vi "Waveform Envelope.vi"() -> ()   [LabVIEW 2020]
panel:
  out "From Origin":dynamicdata(graph)
  in  "Visible":i32(ring) items=["MAINWND_HIDE"=0, "MAINWND_SHOW"=1, "MAINWND_SHOWMINIMIZED"=2, "MAINWND_SHOWMAXIMIZED"=3, "MAINWND_SHOW_BRING_TO_FRONT"=100]
  out "data filepath":path
  in  "GetEnvelope":bool
  out "ogw path":path
  out "Origin ogw Load":bool
  out "Error Out":errorcluster
  out "Input Data":waveform(dbl)(graph)
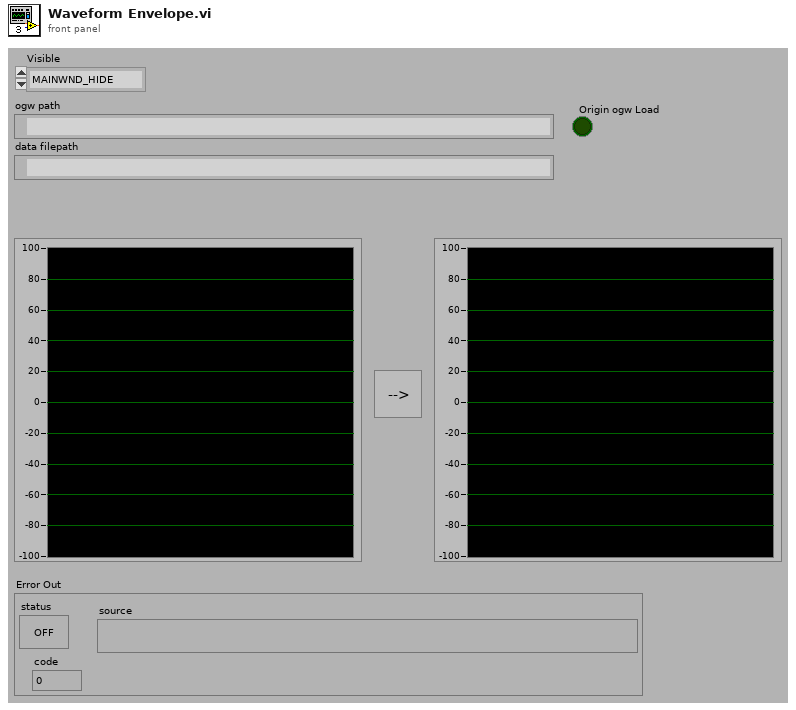
[diagram p1: front panel]
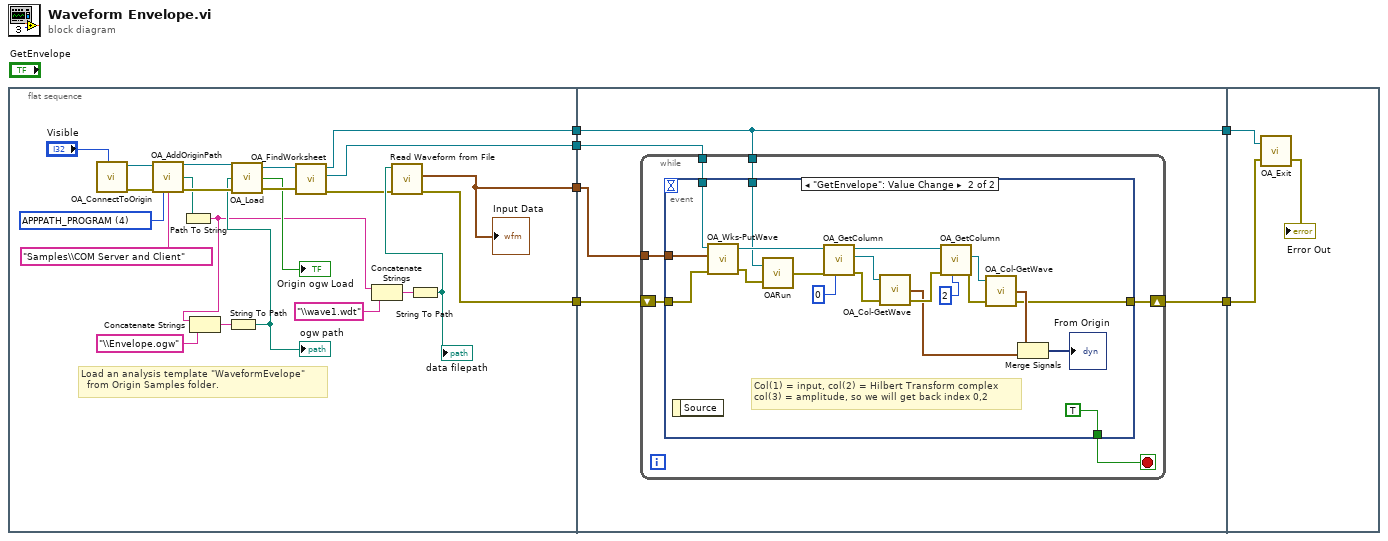
[diagram p0: block diagram]
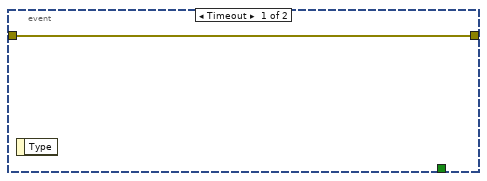
[diagram p2: hidden frame]
diagram:
  n1 = flat-sequence {
    tunnel: [w10] -> w6
    tunnel: [w9] -> w5
    tunnel: [w8] -> w4
    tunnel: [w7] -> w2
    tunnel: w6 -> [w34]
    tunnel: w5 -> [w32]
    tunnel: w4 -> [w33]
    tunnel: [w32] -> w3
    tunnel: w2 -> [w31]
    tunnel: [w30] -> w1
    tunnel: w3 -> [w63]
    tunnel: w1 -> [w62]
    frame #0 {
      w27 = 4 items=["APPPATH_USER"=2, "APPPATH_GROUP"=3, "APPPATH_PROGRAM"=4] ("Type")
      # "Load an analysis template \"WaveformEvelope\"\n  from Origin Samples folder."
      n2 = call "OA_ConnectToOrigin.vi"("Visible"="Visible") -> ("error out"=w22:errorcluster, "Origin.IOApplication"=w23:refnum<k7>)  [unwired: 7 in]
      n3 = call "OA_AddOriginPath.vi"("Origin.IOApplication"=w23, "error in (no error)"=w22, "Type"=w27, "Filename"="Samples\\COM Server and Client") -> ("Origin.IOApplication"=w29:refnum<k7>, "path out"=w17:path, "error out"=w28:errorcluster)  [unwired: 9 in]
      n4 = Path To String(path=w17) -> (string=w11:string)
      n5 = Concatenate Strings(w11, "\\Envelope.ogw" ("string")) -> (w19:string)
      n6 = String To Path(string=w19) -> (path=w18:path)
      "ogw path" <- w18
      n7 = call "OA_Load.vi"("error in (no error)"=w28, "Path"=w18, "Origin.IOApplication"=w29) -> ("error out"=w24:errorcluster, "Load"=→"Origin ogw Load":bool, "Origin.IOApplication"=w25:refnum<k7>)
      n8 = call "OA_FindWorksheet.vi"("error in (no error)"=w24, "Origin.IOApplication"=w25) -> ("error out"=w12:errorcluster, "Origin.Worksheet"=w8:refnum<k7>, "Origin.IOApplication"=w9:refnum<k7>)  [unwired: 7 in]
      n9 = Concatenate Strings(w11, "\\wave1.wdt" ("string")) -> (w14:string)
      n10 = String To Path(string=w14) -> (path=w15:path)
      "data filepath" <- w15
      n11 = call <vilib>:"Read Waveform from File.vi"("error in (no error)"=w12, "file path (dialog if empty)"=w15) -> ("error out"=w7:errorcluster, "first waveform in record"=w10:waveform(dbl))  [unwired: 4 in, 2 out]
      "Input Data" <- w10
    }
    frame #1 {
      n12 = while {
        tunnel: w34 -> [w40]
        tunnel: w33 -> [w39]
        tunnel: w32 -> [w38]
        shift-right: [w36] -> w30
        shift-left: w31 -> [w37]
        stop <- w35 stop-if-true
        n13 = event shown="[1] \"GetEnvelope\": Value Change" {
          selector: _ -> [_ _]
          dyn-events: _ -> [_ _]
          timeout: _ -> [_ _]
          tunnel: w40 -> [_ w49]
          tunnel: w39 -> [_ w48]
          tunnel: w38 -> [_ w47]
          tunnel: w37 -> [w41 w46]
          tunnel: [w41 w42] -> w36
          tunnel: [_ TRUE] -> w35
          event Timeout {
            n14 = event-data() -> ()  [unwired: 1 in, 1 out]
          }
          event "GetEnvelope": Value Change {
            # "Col(1) = input, col(2) = Hilbert Transform complex\ncol(3) = amplitude, so we will get back index 0,2"
            n15 = event-data() -> ()  [unwired: 1 in, 1 out]
            n16 = call "OA_Wks-PutWave.vi"("Origin.Worksheet"=w48, "Dynamic Data"=w49, "error in (no error)"=w46) -> ("Origin.Worksheet dup"=w59:refnum<k7>, "error IO"=w60:errorcluster)  [unwired: 3 in]
            n17 = call "OARun.vi"("Origin.IOApplication"=w47, "Error IO"=w60) -> ("Error IO Out"=w61:errorcluster)  [unwired: 2 out]
            n18 = call "OA_GetColumn.vi"("Column Name/Index"=0, "error in (no error)"=w61, "Origin.Worksheet"=w59) -> ("error out"=w56:errorcluster, "Origin.Column"=w43:refnum<k7>, "Origin.Worksheet"=w50:refnum<k7>)  [unwired: 6 in]
            n19 = call "OA_Col-GetWave.vi"("error in (no error)"=w56, "Origin.Column"=w43) -> ("error out"=w53:errorcluster, "Waveform Out"=w52:waveform(dbl))  [unwired: 1 in, 1 out]
            n20 = call "OA_GetColumn.vi"("Column Name/Index"=2, "error in (no error)"=w53, "Origin.Worksheet"=w50) -> ("error out"=w54:errorcluster, "Origin.Column"=w55:refnum<k7>)  [unwired: 6 in, 1 out]
            n21 = call "OA_Col-GetWave.vi"("error in (no error)"=w54, "Origin.Column"=w55) -> ("error out"=w42:errorcluster, "Waveform Out"=w51:waveform(dbl))  [unwired: 1 in, 1 out]
            n22 = Merge Signals(w51, w52) -> (→"From Origin":dynamicdata)
          }
        }
      }
    }
    frame #2 {
      n23 = call "OA_Exit.vi"("Error IO"=w62, "Origin.IOApplication"=w63) -> ("Error IO Out"=→"Error Out":errorcluster)  [unwired: 1 out]
    }
  }
